vi "Load Becker-Hickl File Information.vi"(8 "Error In":errorcluster, 11 "File Path Control":path) -> (0 "Error Out":errorcluster, 2 "Size (in Bytes)":i64, 3 "B&H File Information":T1 {"Measurement Information"."Measurement FCS Info"."FCS Type" format="%016.0f"; "Measurement Information"."Measurement FCS Info"."FCS Decay Calc" format="%016b"; "Measurement Information"."Measurement Stop Info"."Flags" format="%016b"}, 4 "Load Time (s)":dbl)   [LabVIEW 2021, in "Becker-Hickl Files.lvlib"]
uses:
  Becker-Hickl Files.lvlib
  Becker-Hickl File Information.ctl
  Becker-Hickl File Header Structure.ctl
  Becker-Hickl Image Parameters.ctl
  Becker-Hickl TAC Parameters.ctl
  Becker-Hickl Measurement Information.ctl
  Becker-Hickl Measurement Stop Info.ctl
  Becker-Hickl FCS Measurement Info.ctl
  Becker-Hickl Additional Histogram Measurement Info.ctl
  Time/Time.lvlib
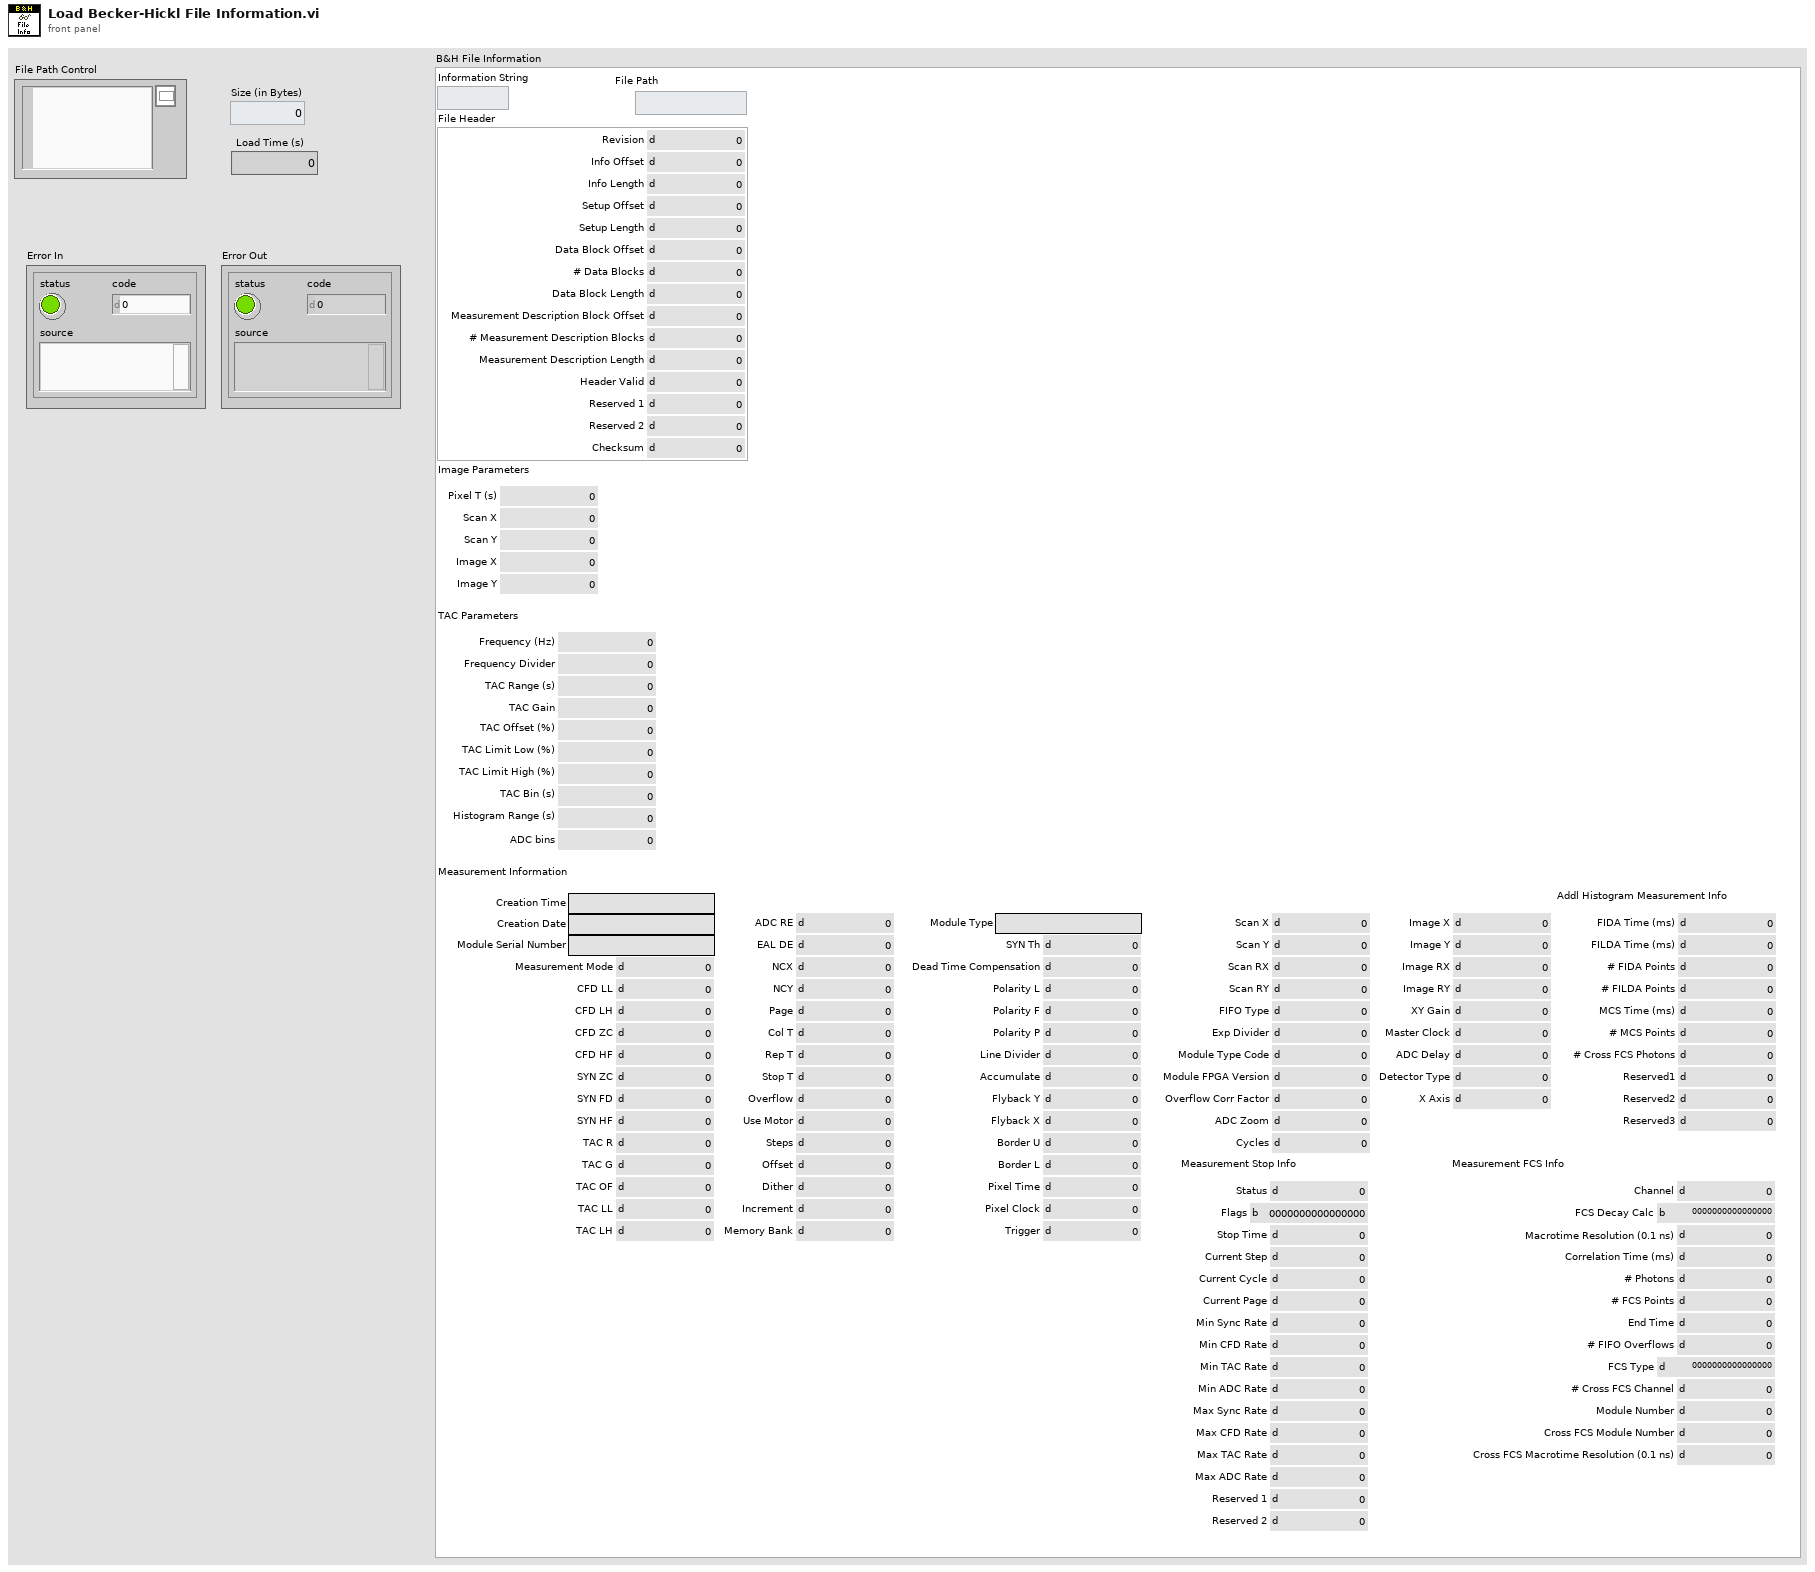
[diagram p1: front panel]
types:
  T1 = typedef "Becker-Hickl Files.lvlib/Becker-Hickl File Information.ctl" = cluster{"Information String":string, "File Header":T2, "Image Parameters":T3, "TAC Parameters":T4, "Measurement Information":T5, "File Path":path}
  T2 = typedef "Becker-Hickl Files.lvlib/Becker-Hickl File Header Structure.ctl" = cluster{"Revision":i16, "Info Offset":i32, "Info Length":i16, "Setup Offset":i32, "Setup Length":i16, "Data Block Offset":i32, "# Data Blocks":i16, "Data Block Length":i32, "Measurement Description Block Offset":i32, "# Measurement Description Blocks":i16, "Measurement Description Length":i16, "Header Valid":u16, "Reserved 1":u32, "Reserved 2":u16, "Checksum":u16}
  T3 = typedef "Becker-Hickl Files.lvlib/Becker-Hickl Image Parameters.ctl" = cluster{"Pixel T (s)":dbl, "Scan X":i32, "Scan Y":i32, "Image X":i32, "Image Y":i32}
  T4 = typedef "Becker-Hickl Files.lvlib/Becker-Hickl TAC Parameters.ctl" = cluster{"Frequency (Hz)":dbl, "Frequency Divider":i32, "TAC Range (s)":dbl, "TAC Gain":i32, "TAC Offset (%)":dbl, "TAC Limit Low (%)":dbl, "TAC Limit High (%)":dbl, "TAC Bin (s)":dbl, "ADC bins":i32, "Histogram Range (s)":dbl}
  T5 = typedef "Becker-Hickl Files.lvlib/Becker-Hickl Measurement Information.ctl" = cluster{"Measurement Stop Info":T6, "Measurement FCS Info":T7, "Addl Histogram Measurement Info":T8, "Creation Time":string, "Creation Date":string, "Module Serial Number":string, "Measurement Mode":i16, "CFD LL":sgl, "CFD LH":sgl, "CFD ZC":sgl, "CFD HF":sgl, "SYN ZC":sgl, "SYN FD":i16, "SYN HF":sgl, "TAC R":sgl, "TAC G":i16, "TAC OF":sgl, "TAC LL":sgl, "TAC LH":sgl, "ADC RE":i16, "EAL DE":i16, "NCX":i16, "NCY":i16, "Page":u16, "Col T":sgl, "Rep T":sgl, "Stop T":i16, "Overflow":u8, "Use Motor":i16, "Steps":u16, "Offset":sgl, "Dither":i16, "Increment":i16, "Memory Bank":i16, "Module Type":string, "SYN Th":sgl, "Dead Time Compensation":i16, "Polarity L":i16, "Polarity F":i16, "Polarity P":i16, "Line Divider":i16, "Accumulate":i16, "Flyback Y":i32, "Flyback X":i32, "Border U":i32, "Border L":i32, "Pixel Time":sgl, "Pixel Clock":i16, "Trigger":i16, "Scan X":i32, "Scan Y":i32, "Scan RX":i32, "Scan RY":i32, "FIFO Type":i16, "Exp Divider":i32, "Module Type Code":u16, "Module FPGA Version":u16, "Overflow Corr Factor":sgl, "ADC Zoom":i32, "Cycles":i32, "Image X":i32, "Image Y":i32, "Image RX":i32, "Image RY":i32, "XY Gain":i16, "Master Clock":i16, "ADC Delay":i16, "Detector Type":i16, "X Axis":i16}
  T6 = typedef "Becker-Hickl Files.lvlib/Becker-Hickl Measurement Stop Info.ctl" = cluster{"Status":u16, "Flags":u16, "Stop Time":sgl, "Current Step":i32, "Current Cycle":i32, "Current Page":i32, "Min Sync Rate":sgl, "Min CFD Rate":sgl, "Min TAC Rate":sgl, "Min ADC Rate":sgl, "Max Sync Rate":sgl, "Max CFD Rate":sgl, "Max TAC Rate":sgl, "Max ADC Rate":sgl, "Reserved 1":i32, "Reserved 2":sgl}
  T7 = typedef "Becker-Hickl Files.lvlib/Becker-Hickl FCS Measurement Info.ctl" = cluster{"Channel":u16, "FCS Decay Calc":u16, "Macrotime Resolution (0.1 ns)":u32, "Correlation Time (ms)":sgl, "# Photons":u32, "# FCS Points":i32, "End Time":sgl, "# FIFO Overflows":u16, "FCS Type":u16, "# Cross FCS Channel":u16, "Module Number":u16, "Cross FCS Module Number":u16, "Cross FCS Macrotime Resolution (0.1 ns)":u32}
  T8 = typedef "Becker-Hickl Files.lvlib/Becker-Hickl Additional Histogram Measurement Info.ctl" = cluster{"FIDA Time (ms)":sgl, "FILDA Time (ms)":sgl, "# FIDA Points":i32, "# FILDA Points":i32, "MCS Time (ms)":sgl, "# MCS Points":i32, "# Cross FCS Photons":u32, "Reserved1":i32, "Reserved2":dbl, "Reserved3":dbl}
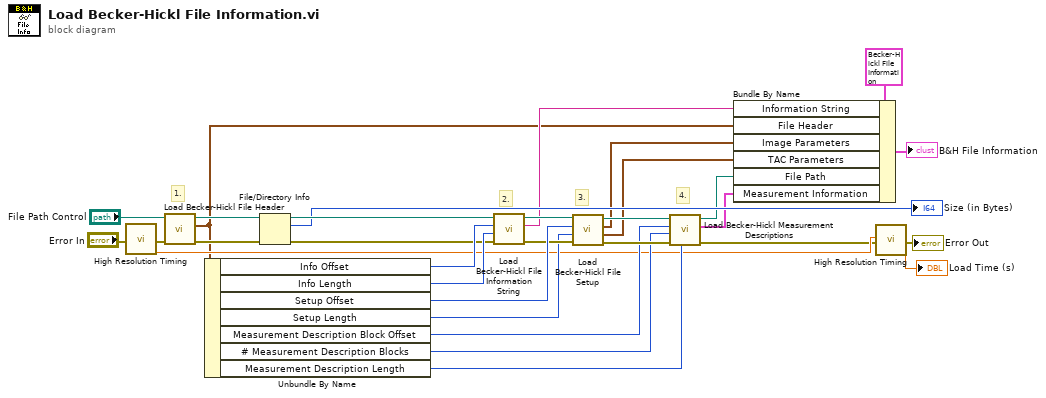
[diagram p0: block diagram]
diagram:
  # "4."
  # "1."
  # "3."
  # "2."
  n1 = call "High Resolution Timing.vi"("Error In"="Error In") -> ("elapsed (relative) seconds"=w11:dbl, "Error Out"=w13:errorcluster)  [unwired: 16 in, 1 out]
  n2 = call "Load Becker-Hickl File Header.vi"("Error In"=w13, "File Path Control"="File Path Control") -> ("Error Out"=w16:errorcluster, "B& H File Header"=w8:T2, "File Path out"=w31:path)  [unwired: 7 in]
  n3 = Unbundle By Name(w8) -> ("Info Offset"=w28:i32, "Info Length"=w27:i16, "Setup Offset"=w26:i32, "Setup Length"=w23:i16, "Measurement Description Block Offset"=w20:i32, "# Measurement Description Blocks"=w19:i16, "Measurement Description Length"=w18:i16)
  n4 = File/Directory Info(path=w31, error in=w16) -> (path out=w17:path, size=→"Size (in Bytes)":i64, error out=w15:errorcluster)  [unwired: 4 out]
  n5 = call "Load Becker-Hickl File Information String.vi"("Error In"=w15, "Info Length"=w27, "Info Offset"=w28, "File Path in"=w17) -> ("Error Out"=w24:errorcluster, "Information String"=w9:string, "File Path out"=w25:path)  [unwired: 5 in]
  n6 = call "Load Becker-Hickl File Setup.vi"("Error In"=w24, "Setup Length"=w23, "Setup Offset"=w26, "File Path Control"=w25) -> ("Error Out"=w21:errorcluster, "TAC Parameters"=w6:T4, "Image Parameters"=w7:T3, "File Path out"=w22:path)  [unwired: 3 in, 1 out]
  n7 = call "Load Becker-Hickl Measurement Descriptions.vi"("Measurement Description Length"=w18, "Error In"=w21, "# Measurement Description Blocks"=w19, "Measurement Description Block Offset"=w20, "File Path Control"=w22) -> ("Error Out"=w3:errorcluster, "Measurement Information"=w1:T5, "File Path"=w2:path)  [unwired: 4 in]
  n8 = Bundle By Name(cluster=T1 {"Information String"="", "File Header"={"Revision"=0, "Info Offset"=0, "Info Length"=0, "Setup Offset"=0, "Setup Length"=0, "Data Block Offset"=0, "# Data Blocks"=0, "Data Block Length"=0, "Measurement Description Block Offset"=0, "# Measurement Description Blocks"=0, "Measurement Description Length"=0, "Header Valid"=0, "Reserved 1"=0, "Reserved 2"=0, "Checksum"=0}, "Image Parameters"={"Pixel T (s)"=0.0, "Scan X"=0, "Scan Y"=0, "Image X"=0, "Image Y"=0}, "TAC Parameters"={"Frequency (Hz)"=0.0, "Frequency Divider"=0, "TAC Range (s)"=0.0, "TAC Gain"=0, "TAC Offset (%)"=0.0, "TAC Limit Low (%)"=0.0, "TAC Limit High (%)"=0.0, "TAC Bin (s)"=0.0, "ADC bins"=0, "Histogram Range (s)"=0.0}, "Measurement Information"={"Measurement Stop Info"={"Status"=0, "Flags"=0, "Stop Time"=0.0, "Current Step"=0, "Current Cycle"=0, "Current Page"=0, "Min Sync Rate"=0.0, "Min CFD Rate"=0.0, "Min TAC Rate"=0.0, "Min ADC Rate"=0.0, "Max Sync Rate"=0.0, "Max CFD Rate"=0.0, "Max TAC Rate"=0.0, "Max ADC Rate"=0.0, "Reserved 1"=0, "Reserved 2"=0.0}, "Measurement FCS Info"={"Channel"=0, "FCS Decay Calc"=0, "Macrotime Resolution (0.1 ns)"=0, "Correlation Time (ms)"=0.0, "# Photons"=0, "# FCS Points"=0, "End Time"=0.0, "# FIFO Overflows"=0, "FCS Type"=0, "# Cross FCS Channel"=0, "Module Number"=0, "Cross FCS Module Number"=0, "Cross FCS Macrotime Resolution (0.1 ns)"=0}, "Addl Histogram Measurement Info"={"FIDA Time (ms)"=0.0, "FILDA Time (ms)"=0.0, "# FIDA Points"=0, "# FILDA Points"=0, "MCS Time (ms)"=0.0, "# MCS Points"=0, "# Cross FCS Photons"=0, "Reserved1"=0, "Reserved2"=0.0, "Reserved3"=0.0}, "Creation Time"="", "Creation Date"="", "Module Serial Number"="", "Measurement Mode"=0, "CFD LL"=0.0, "CFD LH"=0.0, "CFD ZC"=0.0, "CFD HF"=0.0, "SYN ZC"=0.0, "SYN FD"=0, "SYN HF"=0.0, "TAC R"=0.0, "TAC G"=0, "TAC OF"=0.0, "TAC LL"=0.0, "TAC LH"=0.0, "ADC RE"=0, "EAL DE"=0, "NCX"=0, "NCY"=0, "Page"=0, "Col T"=0.0, "Rep T"=0.0, "Stop T"=0, "Overflow"=0, "Use Motor"=0, "Steps"=0, "Offset"=0.0, "Dither"=0, "Increment"=0, "Memory Bank"=0, "Module Type"="", "SYN Th"=0.0, "Dead Time Compensation"=0, "Polarity L"=0, "Polarity F"=0, "Polarity P"=0, "Line Divider"=0, "Accumulate"=0, "Flyback Y"=0, "Flyback X"=0, "Border U"=0, "Border L"=0, "Pixel Time"=0.0, "Pixel Clock"=0, "Trigger"=0, "Scan X"=0, "Scan Y"=0, "Scan RX"=0, "Scan RY"=0, "FIFO Type"=0, "Exp Divider"=0, "Module Type Code"=0, "Module FPGA Version"=0, "Overflow Corr Factor"=0.0, "ADC Zoom"=0, "Cycles"=0, "Image X"=0, "Image Y"=0, "Image RX"=0, "Image RY"=0, "XY Gain"=0, "Master Clock"=0, "ADC Delay"=0, "Detector Type"=0, "X Axis"=0}, "File Path"=path ""} ("output cluster"), "Information String"=w9, "File Header"=w8, "Image Parameters"=w7, "TAC Parameters"=w6, "File Path"=w2, "Measurement Information"=w1) -> (→"B&H File Information":T1)
  n9 = call "High Resolution Timing.vi"("relative seconds (NaN)"=w11, "Error In"=w3) -> ("elapsed (relative) seconds"=→"Load Time (s)":dbl, "Error Out"=→"Error Out":errorcluster)  [unwired: 15 in, 1 out]
